vi "HF AccUView.vi"(4 "State":i16, 5 "Time":dbl format="%.2f", 6 "Sensor Values":dbl[](array[numeric]), 7 "Set Points":dbl[](array[numeric])=[1.0]) -> (0 "required data":T2={"Set Point names"=["data interval (s)", "com port number", "device ID", "register address"], "required number of setpoints"=4, "required number of sensors"=0, "Sensor names"=[]}, 3 "output value":dbl)   [LabVIEW 2019]
panel:
  in  "Parity":u16(ring)=2 items=["None", "Odd", "Even", "Mark", "Space"]
  in  "set point inputs":T1
  out "error out":errorcluster
  out "VISA resource name out":refnum<visa-resource-name>
  in  "error in (no error)":errorcluster
  # "Enter the correct information for this control code in the required data structure below. Then make the current value default by right clicking on the border of the data structure. Select \"data operations\" and then select \"make current value default\". These values will be displayed by process controller."
  # "HF turbidimeters have none for parity as default.\nNeed to change to Even!"
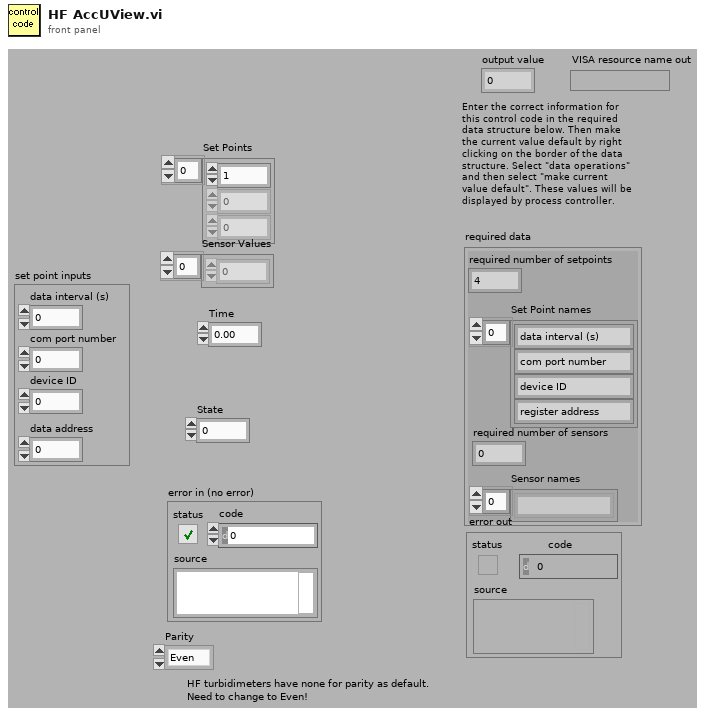
[diagram p1: front panel]
types:
  T1 = cluster{"data interval (s)":dbl, "com port number":u8, "device ID":u8, "data address":u8}
  T2 = cluster{"Set Point names":string[], "required number of setpoints":u8, "required number of sensors":u8, "Sensor names":string[]}
  T3 = cluster{"Set Points[0]":dbl, "Set Points[1]":dbl, "Set Points[2]":dbl, "Set Points[3]":dbl}
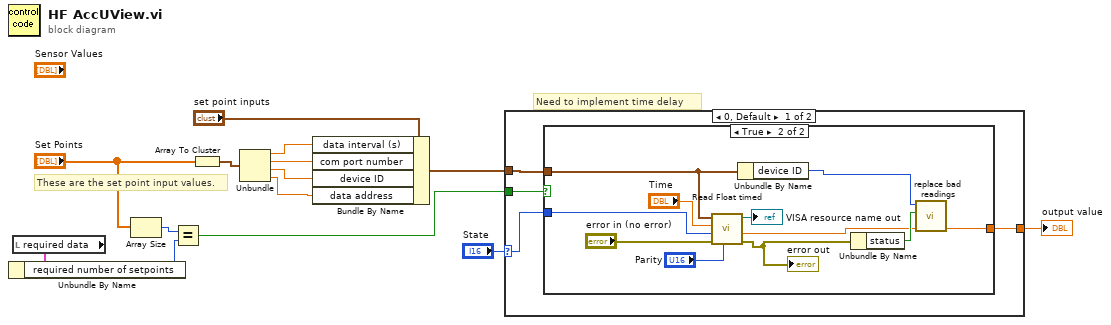
[diagram p0: block diagram]
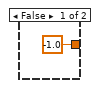
[diagram p2: hidden frame]
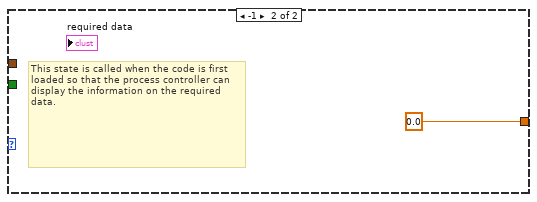
[diagram p3: hidden frame]
diagram:
  # "Need to implement time delay"
  # "These are the set point input values."
  n1 = local read "required data"() -> (w4:T2)
  n2 = Unbundle By Name(w4) -> ("required number of setpoints"=w3:u8)
  n3 = Array Size(array="Set Points") -> (size(s)=w5:i32)
  n4 = Equal?(x=w5, y=w3) -> (x = y?=w2:bool)
  n5 = Array To Cluster(array="Set Points") -> (cluster=w11:T3)
  n6 = Unbundle(w11) -> ("Set Points[0]"=w10:dbl, "Set Points[1]"=w12:dbl, "Set Points[2]"=w9:dbl, "Set Points[3]"=w1:dbl)
  n7 = Bundle By Name(cluster="set point inputs", "data interval (s)"=w10, "com port number"=w12, "device ID"=w9, "data address"=w1) -> (w8:T1)
  n8 = case shown="0, Default" "State" {
    selector: "State" -> [w16 _]
    tunnel: [w17 0.0 ("fraction on")] -> w13
    tunnel: w8 -> [w18 _]
    tunnel: w2 -> [w15 _]
    frame 0, Default {
      n9 = case shown="True" w15 {
        tunnel: w18 -> [_ w28]
        tunnel: [-1.0 ("Meter reading out") w26] -> w17
        tunnel: w16 -> [_ w22]
        frame False {
        }
        frame True {
          n10 = call "Read Float timed.vi"("Parity"="Parity", "error in"="error in (no error)", "State"=w22, "Time"="Time", "set point inputs"=w28) -> ("error out"=w20:errorcluster, "output value"=w29:dbl, "VISA resource name out"=→"VISA resource name out":refnum<visa-resource-name>)  [unwired: 3 in, 1 out]
          "error out" <- w20
          n11 = Unbundle By Name(w28) -> ("device ID"=w27:u8)
          n12 = Unbundle By Name(w20) -> ("status"=w30:bool)
          n13 = call "replace bad readings.vi"("Meter reading in"=w29, "bad data read"=w30, "Unit ID"=w27) -> ("Meter reading out"=w26:dbl)  [unwired: 8 in]
        }
      }
    }
    frame -1 {
      # "This state is called when the code is first loaded so that the process controller can display the information on the required data."
    }
  }
  "output value" <- w13
